vi "PH_gentec_M-Link.ProcEvents.vi"(0 "i ref in":refnum<vi>, 5 "error in":errorcluster) -> (14 "i ref out":refnum<vi>, 19 "error out":errorcluster)   [LabVIEW 2014, in "PH_gentec_M-Link.lvlib"]
doc: "This method is used to define the events the object will listen to. Add your own events here."
uses:
  PH_gentec_M-Link.lvlib
  CS_Core/BaseProcess/BaseProcess.event definition.ctl
  CS_Core/CAEObj/CAEObj.event definition.ctl
  CS_Core/BaseProcess/BaseProcess.descriptor string definition.ctl
  CS_Core/BaseProcess/BaseProcess.lvlib
  CS_Core/CAEObj/CAEObj.lvlib
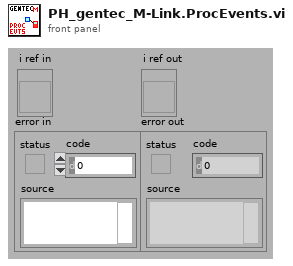
[diagram p1: front panel]
types:
  T1 = typedef "BaseProcess.lvlib/BaseProcess.event definition.ctl" = cluster{"CAEEvtDef":T2, "Data Descriptor":T3}
  T2 = typedef "CAEObj.lvlib/CAEObj.event definition.ctl" = cluster{"URL":string, "enable":bool, "ignoreResID":bool}
  T3 = typedef "BaseProcess.lvlib/BaseProcess.descriptor string definition.ctl" = string
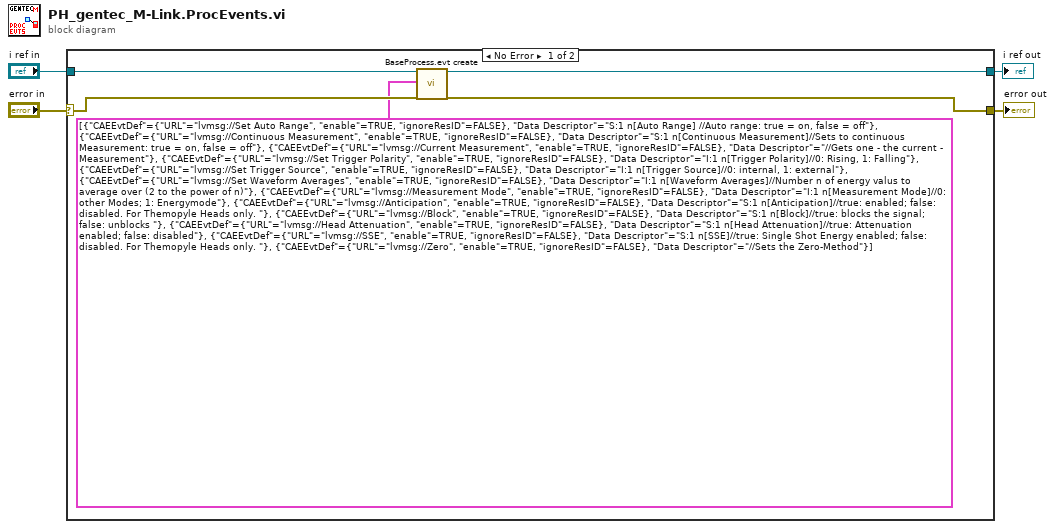
[diagram p0: block diagram]
diagram:
  n1 = case shown="No Error" "error in" {
    selector: "error in" -> [w7 w10]
    tunnel: "i ref in" -> [w6 w11]
    tunnel: [w9 w11] -> w3
    tunnel: [w8 w10] -> w2
    frame No Error {
      n2 = call "BaseProcess.evt create.vi"("i ref in"=w6, "newEvents"=T1[] [{"CAEEvtDef"={"URL"="lvmsg://Set Auto Range", "enable"=TRUE, "ignoreResID"=FALSE}, "Data Descriptor"="S:1 n[Auto Range] //Auto range: true = on, false = off"}, {"CAEEvtDef"={"URL"="lvmsg://Continuous Measurement", "enable"=TRUE, "ignoreResID"=FALSE}, "Data Descriptor"="S:1 n[Continuous Measurement]//Sets to continuous Measurement: true = on, false = off"}, {"CAEEvtDef"={"URL"="lvmsg://Current Measurement", "enable"=TRUE, "ignoreResID"=FALSE}, "Data Descriptor"="//Gets one - the current - Measurement"}, {"CAEEvtDef"={"URL"="lvmsg://Set Trigger Polarity", "enable"=TRUE, "ignoreResID"=FALSE}, "Data Descriptor"="I:1 n[Trigger Polarity]//0: Rising, 1: Falling"}, {"CAEEvtDef"={"URL"="lvmsg://Set Trigger Source", "enable"=TRUE, "ignoreResID"=FALSE}, "Data Descriptor"="I:1 n[Trigger Source]//0: internal, 1: external"}, {"CAEEvtDef"={"URL"="lvmsg://Set Waveform Averages", "enable"=TRUE, "ignoreResID"=FALSE}, "Data Descriptor"="I:1 n[Waveform Averages]//Number n of energy valus to average over (2 to the power of n)"}, {"CAEEvtDef"={"URL"="lvmsg://Measurement Mode", "enable"=TRUE, "ignoreResID"=FALSE}, "Data Descriptor"="I:1 n[Measurement Mode]//0: other Modes; 1: Energymode"}, {"CAEEvtDef"={"URL"="lvmsg://Anticipation", "enable"=TRUE, "ignoreResID"=FALSE}, "Data Descriptor"="S:1 n[Anticipation]//true: enabled; false: disabled. For Themopyle Heads only. "}, {"CAEEvtDef"={"URL"="lvmsg://Block", "enable"=TRUE, "ignoreResID"=FALSE}, "Data Descriptor"="S:1 n[Block]//true: blocks the signal; false: unblocks "}, {"CAEEvtDef"={"URL"="lvmsg://Head Attenuation", "enable"=TRUE, "ignoreResID"=FALSE}, "Data Descriptor"="S:1 n[Head Attenuation]//true: Attenuation enabled; false: disabled"}, {"CAEEvtDef"={"URL"="lvmsg://SSE", "enable"=TRUE, "ignoreResID"=FALSE}, "Data Descriptor"="S:1 n[SSE]//true: Single Shot Energy enabled; false: disabled. For Themopyle Heads only. "}, {"CAEEvtDef"={"URL"="lvmsg://Zero", "enable"=TRUE, "ignoreResID"=FALSE}, "Data Descriptor"="//Sets the Zero-Method"}], "error in (no error)"=w7) -> ("i ref out"=w9:refnum<vi>, "error out"=w8:errorcluster)  [unwired: 13 in, 2 out]
    }
    frame Error {
    }
  }
  "i ref out" <- w3
  "error out" <- w2
